vi "Binary to ASCII - Folder Version v2.vi"(8 "error in":errorcluster, 11 "file path (use dialog)":path) -> ()   [LabVIEW 2013]
panel:
  out "error out":errorcluster
  out "Single Fname":string
  out "All Filenames":string[](array[string])
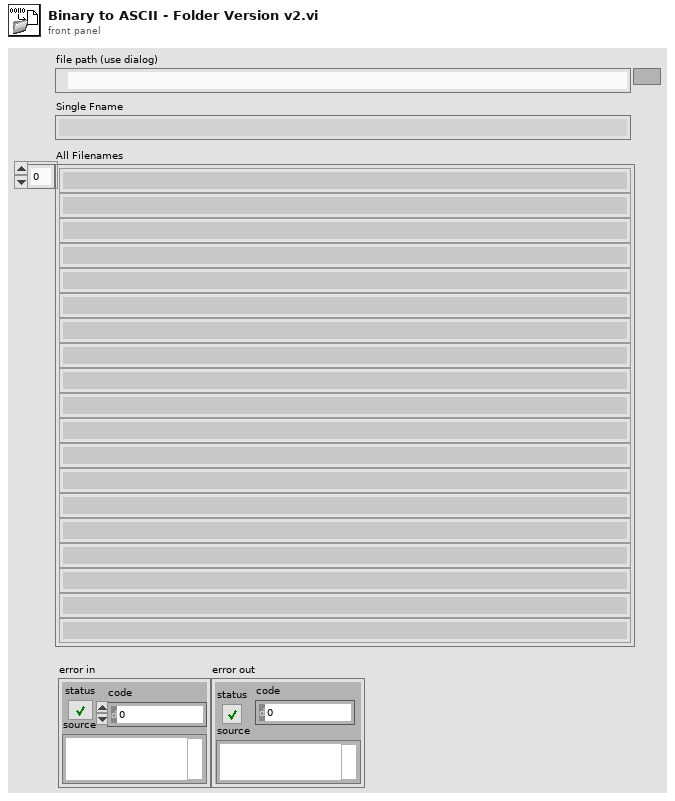
[diagram p1: front panel]
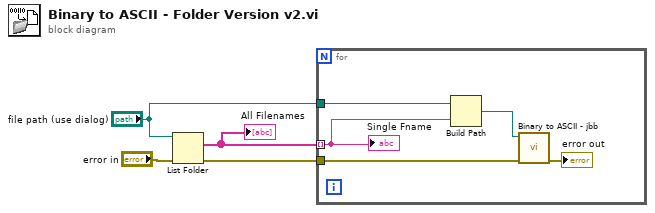
[diagram p0: block diagram]
diagram:
  n1 = List Folder(path="file path (use dialog)", error in="error in") -> (filenames=w1:string[], error out=w3:errorcluster)  [unwired: 2 in, 2 out]
  "All Filenames" <- w1
  n2 = for {
    tunnel: w3 -> [w7]
    tunnel: "file path (use dialog)" -> [w9]
    tunnel: w1 -> [w8] mode=indexing
    n3 = Build Path(base path=w9, name or relative path=w8) -> (appended path=w6:path)
    n4 = call "Binary to ASCII - jbb.vi"("Binary File & Path"=w6, "error in"=w7) -> ("error out"=→"error out":errorcluster)  [unwired: 8 in]
    "Single Fname" <- w8
  }
